vi "GetFlowSensors.vi"(8 "error in (no error)":errorcluster, 10 "Settings in":T2, 11 "refnum":T1) -> (0 "error out":errorcluster, 2 "Settings out":T2, 3 "refnum out":T1)   [LabVIEW 2026]
uses:
  Settings.ctl
  Acquisition/Hardware Configuration.ctl
  Logging/Logging Configuration.ctl
  <vilib>/Utility/config.llb/Config Data RefNum.ctl
  <vilib>/Utility/config.llb/Read Key (String).vi
  <vilib>/Utility/config.llb/NI_LVConfig.lvlib
  Acquisition/Acquisition.lvlib
  Logging/Logging.lvlib
  Settings.lvlib
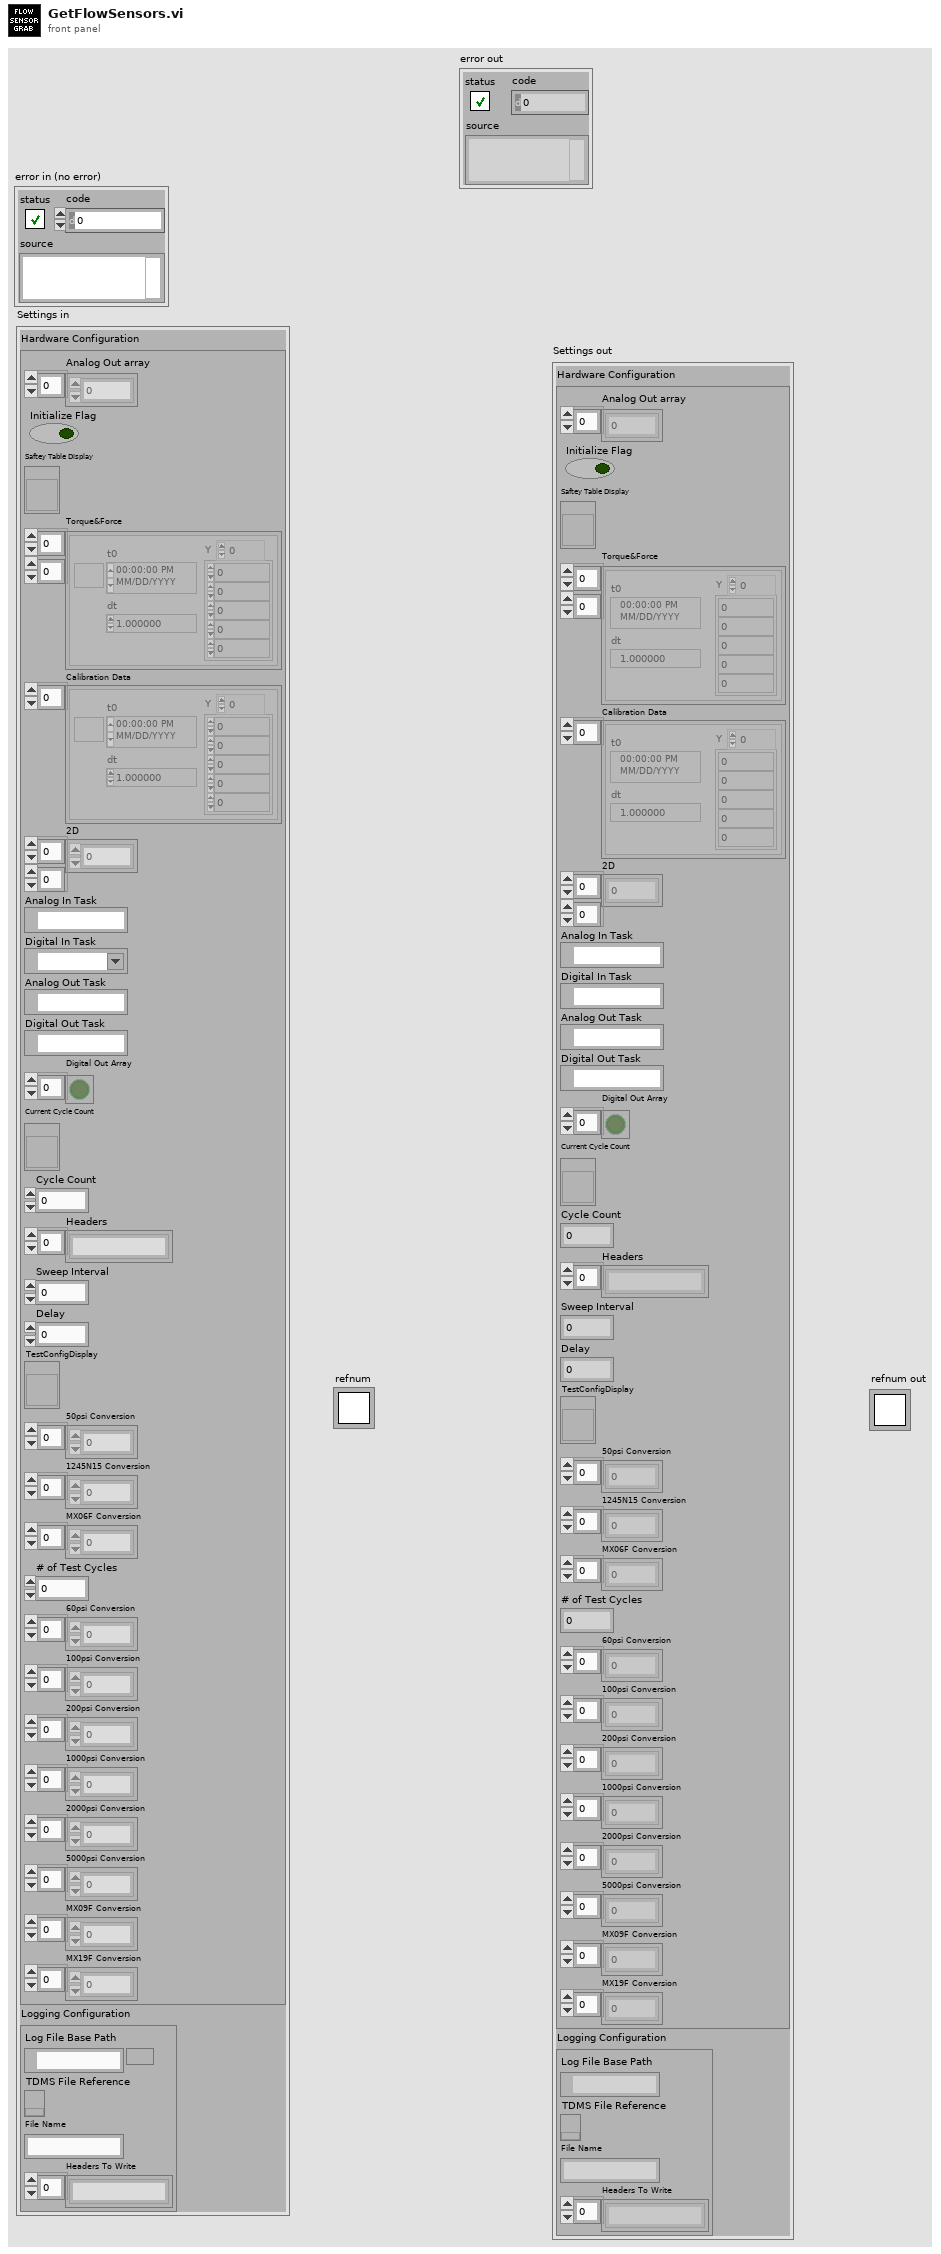
[diagram p1: front panel]
types:
  T1 = typedef "NI_LVConfig.lvlib/Config Data RefNum.ctl" = refnum<k1>
  T2 = typedef "Settings.lvlib/Settings.ctl" = cluster{"Hardware Configuration":T3, "Logging Configuration":T4}
  T3 = typedef "Acquisition.lvlib/Hardware Configuration.ctl" = cluster{"Analog Out array":dbl[], "Initialize Flag":bool, "Saftey Table Display":refnum<vi>, "Torque&Force":waveform(dbl)[][], "Calibration Data":waveform(dbl)[], "2D":dbl[][], "Analog In Task":refnum<k21>, "Digital In Task":refnum<k21>, "Analog Out Task":refnum<k21>, "Digital Out Task":refnum<k21>, "Digital Out Array":bool[], "Current Cycle Count":refnum<vi>, "Cycle Count":u64, "Headers":string[], "Sweep Interval":u64, "Delay":u64, "TestConfigDisplay":refnum<vi>, "50psi Conversion":dbl[], "1245N15 Conversion":dbl[], "MX06F Conversion":dbl[], "# of Test Cycles":u64, "60psi Conversion":dbl[], "100psi Conversion":dbl[], "200psi Conversion":dbl[], "1000psi Conversion":dbl[], "2000psi Conversion":dbl[], "5000psi Conversion":dbl[], "MX09F Conversion":dbl[], "MX19F Conversion":dbl[]}
  T4 = typedef "Logging.lvlib/Logging Configuration.ctl" = cluster{"Log File Base Path":path, "TDMS File Reference":refnum<k34>, "File Name":string, "Headers To Write":string[]}
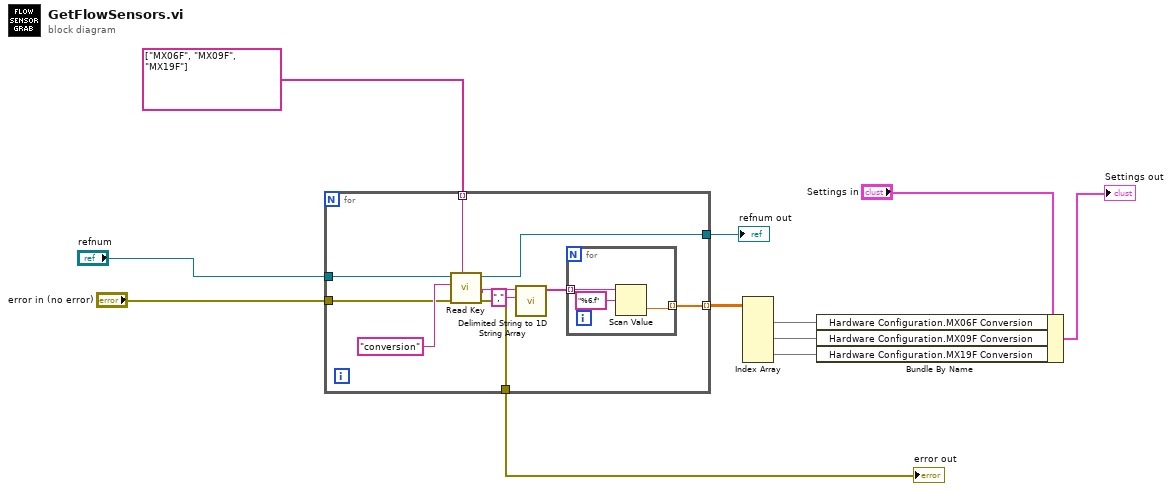
[diagram p0: block diagram]
diagram:
  n1 = for {
    tunnel: string[] ["MX06F", "MX09F", "MX19F"] ("section") -> [w21] mode=indexing
    tunnel: "error in (no error)" -> [w19]
    tunnel: "refnum" -> [w18]
    tunnel: [w14] -> w8 mode=indexing
    tunnel: [w13] -> w2
    tunnel: [w12] -> w1
    n2 = call-poly <vilib>:"Read Key.vi"("section"=w21, "error in (no error)"=w19, "key"="conversion", "refnum"=w18) -> ("error out"=w12:errorcluster, "value"=w15:string, "refnum out"=w13:T1)  [unwired: 4 in, 1 out]
    n3 = call <vilib>:"Delimited String to 1D String Array.vi"("delimiter"=",", "delimited string"=w15) -> ("string array"=w16:string[])  [unwired: 9 in]
    n4 = for {
      tunnel: w16 -> [w24] mode=indexing
      tunnel: [w22] -> w14 mode=indexing
      n5 = Scan Value(string=w24, format string="%6.f") -> (value=w22:dbl)  [unwired: 1 in, 1 out]
    }
  }
  "refnum out" <- w2
  "error out" <- w1
  n6 = Index Array(array=w8) -> (element #1=w7:dbl[], element #2=w6:dbl[], element #3=w5:dbl[])  [unwired: 6 in]
  n7 = Bundle By Name(cluster="Settings in", "Hardware Configuration.MX06F Conversion"=w7, "Hardware Configuration.MX09F Conversion"=w6, "Hardware Configuration.MX19F Conversion"=w5) -> (→"Settings out":T2)
